vi "synnax writer open Array.vi"(4 "start (now)":timestamp, 5 "err_on_unauthorized (F)":bool, 6 "enable_auto_commit (F)":bool, 7 "auto_index (F)":bool, 8 "error in":errorcluster, 9 "authorities (255 for all channels)":u8[](array[numeric]), 10 "channels in":u32[](array[numeric]), 11 "Synnax Client in":refnum<class "Synnax Client.lvclass">) -> (0 "error out":errorcluster, 2 "channels out":u32[](array[numeric]), 3 "writer out":refnum<class "Synnax Writer.lvclass">)   [LabVIEW 2026, in "synnax_clib.lvlib" / "Synnax Writer.lvclass"]
doc: "SYNNAX_EXPORT int32_t synnax_writer_open(\n SynnaxClient client,\n int64_t start,\n const uint32_t *channels,\n uint64_t channel_count,\n int32_t mode,\n int32_t enable_auto_commit,\n SynnaxWriter *out_writer,\n SynnaxError err\n);"
uses:
  Synnax Writer.lvclass
  Client/Synnax Client.lvclass
  Client/Synnax Client.lvclass/Synnax Client.ctl
  Synnax Writer.lvclass/Synnax Writer.ctl
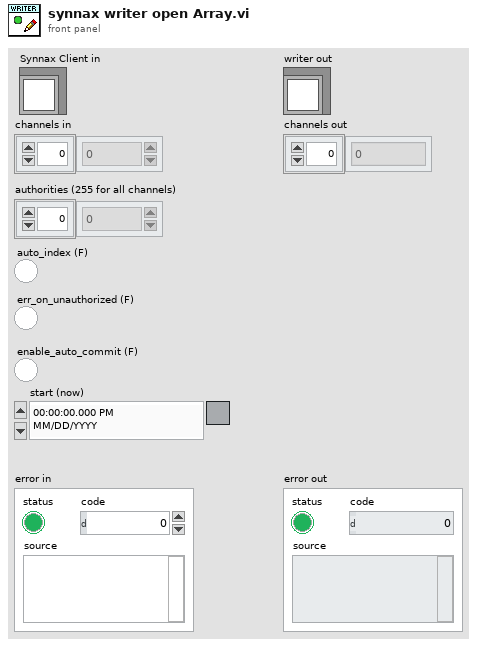
[diagram p1: front panel]
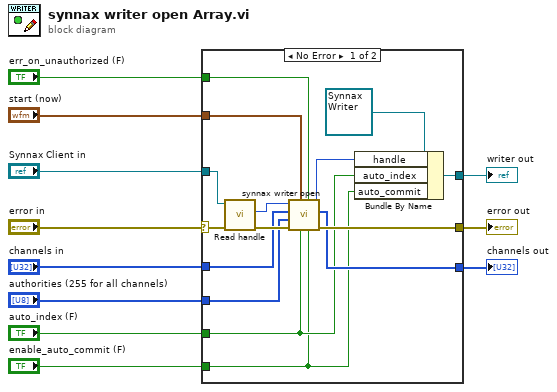
[diagram p0: block diagram]
diagram:
  n1 = case shown="No Error" "error in" {
    selector: "error in" -> [w14 w27]
    tunnel: "Synnax Client in" -> [w26 _]
    tunnel: [w24 _] -> w10
    tunnel: [w23 w27] -> w9
    tunnel: "start (now)" -> [w19 _]
    tunnel: "channels in" -> [w18 _]
    tunnel: "authorities (255 for all channels)" -> [w17 _]
    tunnel: "err_on_unauthorized (F)" -> [w16 _]
    tunnel: "enable_auto_commit (F)" -> [w12 _]
    tunnel: "auto_index (F)" -> [w13 _]
    tunnel: [w15 _] -> w2
    frame No Error {
      n2 = call "Read handle.vi"("error in (no error)"=w14, "Synnax Client in"=w26) -> ("error out"=w20:errorcluster, "handle"=w21:u64)  [unwired: 7 in, 1 out]
      n3 = call "synnax writer open.vi"("enable_auto_commit (F)"=w12, "err_on_unauthorized (F)"=w16, "auto_index (F)"=w13, "start (now)"=w19, "error in"=w20, "authorities (255 for all channels)"=w17, "channels"=w18, "sy client handle"=w21) -> ("error out"=w23:errorcluster, "channels out"=w15:u32[], "sy writer handle"=w22:u64)  [unwired: 1 in]
      n4 = Bundle By Name(cluster=refnum<class "Synnax Writer.lvclass"> refnum, "handle"=w22, "auto_index"=w13, "auto_commit"=w12) -> (w24:refnum<class "Synnax Writer.lvclass">)
    }
    frame Error {
    }
  }
  "error out" <- w9
  "channels out" <- w2
  "writer out" <- w10
